vi "Write receiver.vi"(8 "error in (no error)":errorcluster, 10 "receiver":string, 11 "RxTxCamera in":refnum<class "RxTxCamera.lvclass">) -> (0 "error out":errorcluster, 3 "RxTxCamera out":refnum<class "RxTxCamera.lvclass">)   [LabVIEW 2012, in "RxTxCamera.lvclass"]
uses:
  RxTxCamera.lvclass
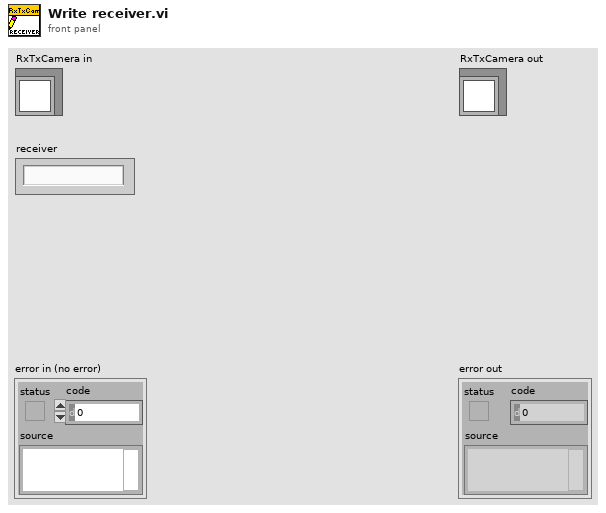
[diagram p1: front panel]
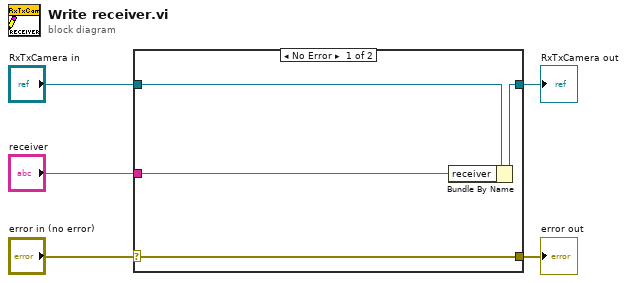
[diagram p0: block diagram]
diagram:
  n1 = case shown="No Error" "error in (no error)" {
    selector: "error in (no error)" -> [w9 w10]
    tunnel: [w9 w10] -> w4
    tunnel: [w7 w11] -> w2
    tunnel: "RxTxCamera in" -> [w8 w11]
    tunnel: "receiver" -> [w6 _]
    frame No Error {
      n2 = Bundle By Name(cluster=w8, "receiver"=w6) -> (w7:refnum<class "RxTxCamera.lvclass">)
    }
    frame Error {
    }
  }
  "error out" <- w4
  "RxTxCamera out" <- w2
